vi "RefNormal_CONVERT.vi"(1 "RefNormal":T5={"Mode"=0, "Fliter"=1, "AccCode"=0, "AccMask"=0, "kBaudRate"=0, "Timing0"=0, "Timing1"=0, "CANRX_EN"=0, "UARTBAUD"=0} {"kBaudRate" items=["SelfDefine", "5 kbps", "10 kbps", "20 kbps", "40 kbps", "50 kbps", "80 kbps", "100 kbps", "125 kbps", "200 kbps", "250 kbps", "400 kbps", "500 kbps", "666 kbps", "800 kbps", "1000 kbps", "33.33 kbps", "66.66 kbps", "83.33 kbps"]; "AccMask" format="%x"; "AccCode" format="%x"; "Fliter" items=["接收所有类型"=1, "只接收标准帧"=2, "只接收扩展帧"=3]; "Mode" items=["正常工作", "仅侦听模式", "自测模式（环回）"]}) -> (0 "RefNormal_1":T1={"Mode"=0, "Fliter"=1, "AccCode 0"=0, "AccCode 1"=0, "AccCode 2"=0, "AccCode 3"=0, "AccMask 0"=0, "AccMask 1"=0, "AccMask 2"=0, "AccMask 3"=0, "kBaudRate"=0, "Timing0"=0, "Timing1"=0, "CANRX_EN"=0, "UARTBAUD"=0} {"AccMask 3" format="%x"; "AccMask 2" format="%x"; "AccMask 1" format="%x"; "AccCode 3" format="%x"; "AccCode 2" format="%x"; "AccCode 1" format="%x"; "kBaudRate" items=["SelfDefine", "5 kbps", "10 kbps", "20 kbps", "40 kbps", "50 kbps", "80 kbps", "100 kbps", "125 kbps", "200 kbps", "250 kbps", "400 kbps", "500 kbps", "666 kbps", "800 kbps", "1000 kbps", "33.33 kbps", "66.66 kbps", "83.33 kbps"]; "AccMask 0" format="%x"; "AccCode 0" format="%x"; "Fliter" items=["接收所有类型"=1, "只接收标准帧"=2, "只接收扩展帧"=3]; "Mode" items=["正常工作", "仅侦听模式", "自测模式（环回）"]})   [LabVIEW 2018, in "ControlCan.lvlib"]
uses:
  ControlCan.lvlib
  RefNormal.ctl
  Mode.ctl
  Fliter.ctl
  kBaudRate.ctl
  RefNormal_1.ctl
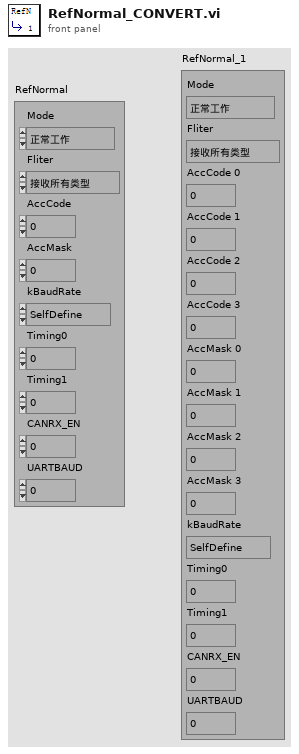
[diagram p1: front panel]
types:
  T1 = typedef "ControlCAN.lvlib/RefNormal_1.ctl" = cluster{"Mode":T2, "Fliter":T3, "AccCode 0":u8, "AccCode 1":u8, "AccCode 2":u8, "AccCode 3":u8, "AccMask 0":u8, "AccMask 1":u8, "AccMask 2":u8, "AccMask 3":u8, "kBaudRate":T4, "Timing0":u8, "Timing1":u8, "CANRX_EN":u8, "UARTBAUD":u8}
  T2 = typedef "ControlCAN.lvlib/Mode.ctl" = u8
  T3 = typedef "ControlCAN.lvlib/Fliter.ctl" = u8
  T4 = typedef "ControlCAN.lvlib/kBaudRate.ctl" = u8
  T5 = typedef "ControlCAN.lvlib/RefNormal.ctl" = cluster{"Mode":T2, "Fliter":T3, "AccCode":u32, "AccMask":u32, "kBaudRate":T4, "Timing0":u8, "Timing1":u8, "CANRX_EN":u8, "UARTBAUD":u8}
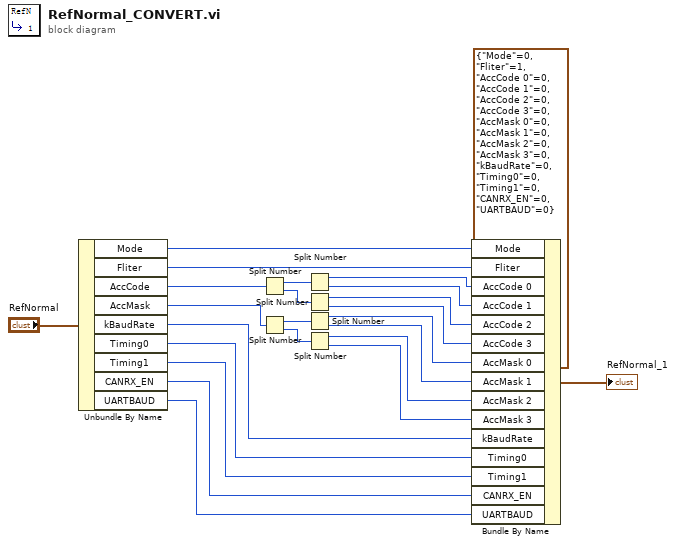
[diagram p0: block diagram]
diagram:
  n1 = Unbundle By Name("RefNormal") -> ("Mode"=w22:T2, "Fliter"=w21:T3, "AccCode"=w20:u32, "AccMask"=w11:u32, "kBaudRate"=w6:T4, "Timing0"=w5:u8, "Timing1"=w4:u8, "CANRX_EN"=w3:u8, "UARTBAUD"=w2:u8)
  n2 = Split Number(x=w20) -> (hi(x)=w19:u16, lo(x)=w18:u16)
  n3 = Split Number(x=w11) -> (hi(x)=w13:u16, lo(x)=w12:u16)
  n4 = Split Number(x=w19) -> (hi(x)=w17:u8, lo(x)=w16:u8)
  n5 = Split Number(x=w18) -> (hi(x)=w15:u8, lo(x)=w14:u8)
  n6 = Split Number(x=w13) -> (hi(x)=w10:u8, lo(x)=w9:u8)
  n7 = Split Number(x=w12) -> (hi(x)=w8:u8, lo(x)=w7:u8)
  n8 = Bundle By Name(cluster=T1 {"Mode"=0, "Fliter"=1, "AccCode 0"=0, "AccCode 1"=0, "AccCode 2"=0, "AccCode 3"=0, "AccMask 0"=0, "AccMask 1"=0, "AccMask 2"=0, "AccMask 3"=0, "kBaudRate"=0, "Timing0"=0, "Timing1"=0, "CANRX_EN"=0, "UARTBAUD"=0} ("RefNormal_1"), "Mode"=w22, "Fliter"=w21, "AccCode 0"=w17, "AccCode 1"=w16, "AccCode 2"=w15, "AccCode 3"=w14, "AccMask 0"=w10, "AccMask 1"=w9, "AccMask 2"=w8, "AccMask 3"=w7, "kBaudRate"=w6, "Timing0"=w5, "Timing1"=w4, "CANRX_EN"=w3, "UARTBAUD"=w2) -> (→"RefNormal_1":T1)
